vi "Set Task List.vi"(8 "error in (no error)":errorcluster, 10 "Task List":refnum<class "Task.lvclass">[](array[class]), 11 "Task Setting Editor in":refnum<class "Task Setting Editor.lvclass">) -> (0 "error out":errorcluster, 3 "Task Setting Editor out":refnum<class "Task Setting Editor.lvclass">)   [LabVIEW 2017, in "Task Setting Editor.lvlib" / "Task Setting Editor.lvclass"]
uses:
  Task Setting Editor.lvclass
  BuildWorker/Classes/Task/Task.lvclass
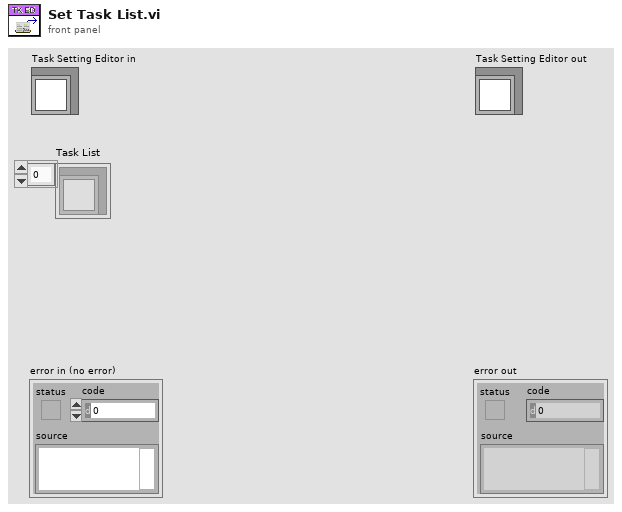
[diagram p1: front panel]
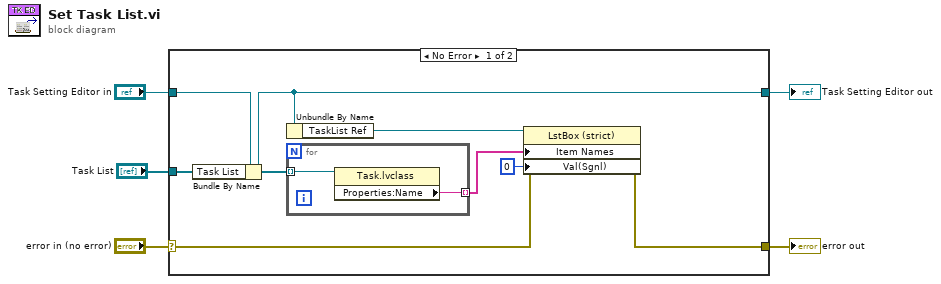
[diagram p0: block diagram]
diagram:
  n1 = case shown="No Error" "error in (no error)" {
    selector: "error in (no error)" -> [w8 w17]
    tunnel: [w7 w17] -> w4
    tunnel: [w11 w16] -> w2
    tunnel: "Task Setting Editor in" -> [w13 w16]
    tunnel: "Task List" -> [w12 _]
    frame No Error {
      n2 = Bundle By Name(cluster=w13, "Task List"=w12) -> (w11:refnum<class "Task Setting Editor.lvclass">)
      n3 = Unbundle By Name(w11) -> ("TaskList Ref"=w10:refnum<vi>)
      n4 = for {
        tunnel: w12 -> [w15] mode=indexing
        tunnel: [w14] -> w9 mode=indexing
        n5 = property class="Task.lvclass"(reference=w15) -> ("Properties:Name"=w14:string)  [unwired: 1 in, 2 out]
      }
      n6 = property class="LstBox (strict)"(reference=w10, error in=w8, "Item Names"=w9, "Val(Sgnl)"=0 ("Value (Signaling)")) -> (error out=w7:errorcluster)  [unwired: 1 out]
    }
    frame Error {
    }
  }
  "error out" <- w4
  "Task Setting Editor out" <- w2
